vi "Begin.vi"(8 "error in":errorcluster) -> (0 "error out":errorcluster)   [LabVIEW 2019]
doc: "Called before other user functions, this VI is expected to open initial I/O refnums, load in file data, and do all program initialization. Notice that the <B>error out</B> terminal is simply used for data flow. Wiring it to other structures or subVIs ensures that this VI runs first."
uses:
  <vilib>/Rock Robotics/WPI/DriverStation/WPI_DriverStationRobotMode2.ctl
  <vilib>/Rock Robotics/WPI/ThirdParty/JAS_Junk/TrajLib/Translation2d_Create.vi
  Robot Global Data.vi
  <vilib>/Rock Robotics/Network Tables/NT Write String Array.vi
  <vilib>/Rock Robotics/WPI/ThirdParty/JAS_Junk/TrajLib/Trajectory_Library.lvlib
panel:
  in  "Tab Control":T1(tab)
  # "Instructions:\nThis should create a path, show the data on the various tabs and optionally write the motor demands and expected results to a file for use on a a robot..\n1) Enter robot data on Robot Data Tab\n2) Define your path definitions.\n3) Define the time increment.  0.020 is chosen since that matches the normal loop time.\n4) Press calculate path.  If a good path was calculated it will be displayed on the Tank Data tab, and the Ready to Execute will indicate execution can begin.\nThe path can be recalculated many times before selecting execute.\n\nTo write to a file.\n5) Select the file name\n6) This example uses \"steps\", sequential numbers for inclusion into a list based autonomous routine.  Including the step number if optional.\n7) This uses command numbers to indicate first, last, and intermediate steps.  This allows some simplification of the execution routine.  It\nalso allows the path to be executed backwards if desired.  The command numbers are changeable.\n8) Press \"Create Command List\".\n\nNotes:\n- PC robot simulataion is disabled in this program.  The code is still there if you want to restore it and try it out.  Use one of the other test programs \nto simulate the path on a PC.\n- The path generation logic doesn't account distribution of speed to the left and right wheels.  As a result the maximum speed can be exceeded.\nIf this happens, but Path Speed > Max light will light and Ready to Execute will not light.  Lower the maximum speed in the Robot Data tab\nand recalulate the path.\n- 2019 playing field size - width: 26 ft 11.25 In = 323.25 in , length: 52 ft 5.25 in = 629.25 in  (I didn't verify this for the 2020 version.)"
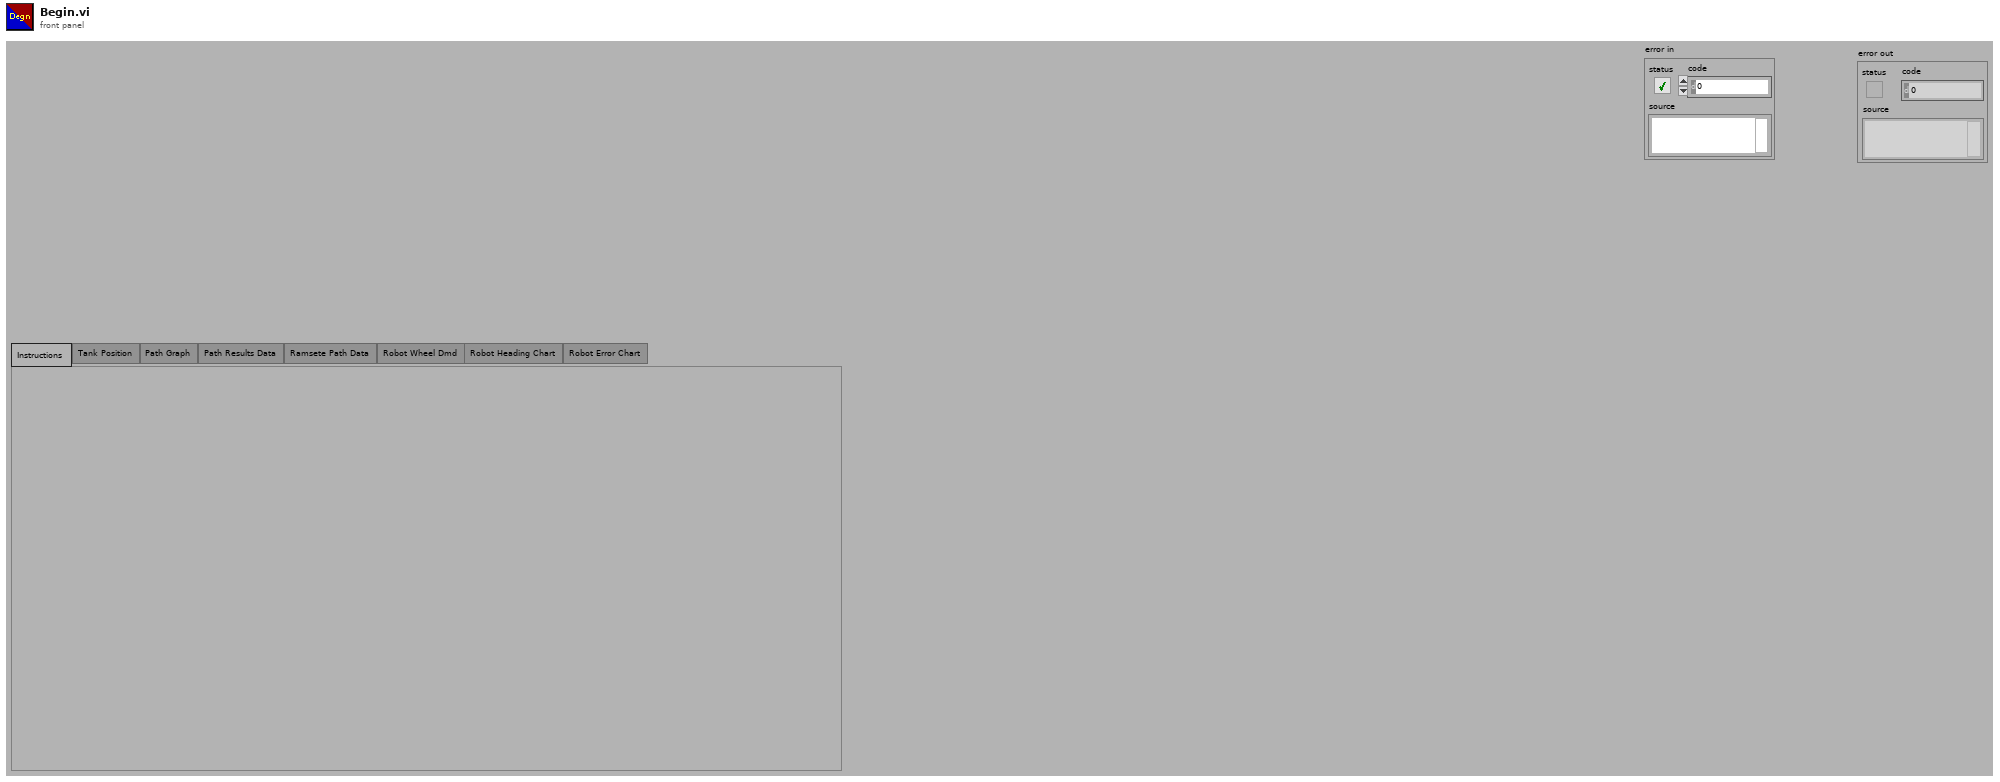
[diagram p1: front panel]
types:
  T1 = enum32{"Instructions", "Tank Position", "Path Graph", "Path Results Data", "Ramsete Path Data", "Robot Wheel Dmd", "Robot Heading Chart", "Robot Error Chart"}
  T2 = typedef "WPI_DriverStationRobotMode2.ctl" = enum16{"Autonomous Disabled", "Autonomous Enabled", "Teleop Disabled", "Teleop Enabled", "Disconnected", "Finish", "Test Disabled", "Test Enabled", "Emergency Stopped"}
  T3 = typedef "Trajectory_Library.lvlib/POSE2D.ctl" = cluster{"TRANSLATION":T4, "ROTATION":T5}
  T4 = typedef "Trajectory_Library.lvlib/TRANSLATION2D.ctl" = cluster{"X":dbl, "Y":dbl}
  T5 = typedef "Trajectory_Library.lvlib/ROTATION2D.ctl" = cluster{"VALUE":dbl, "COS":dbl, "SIN":dbl}
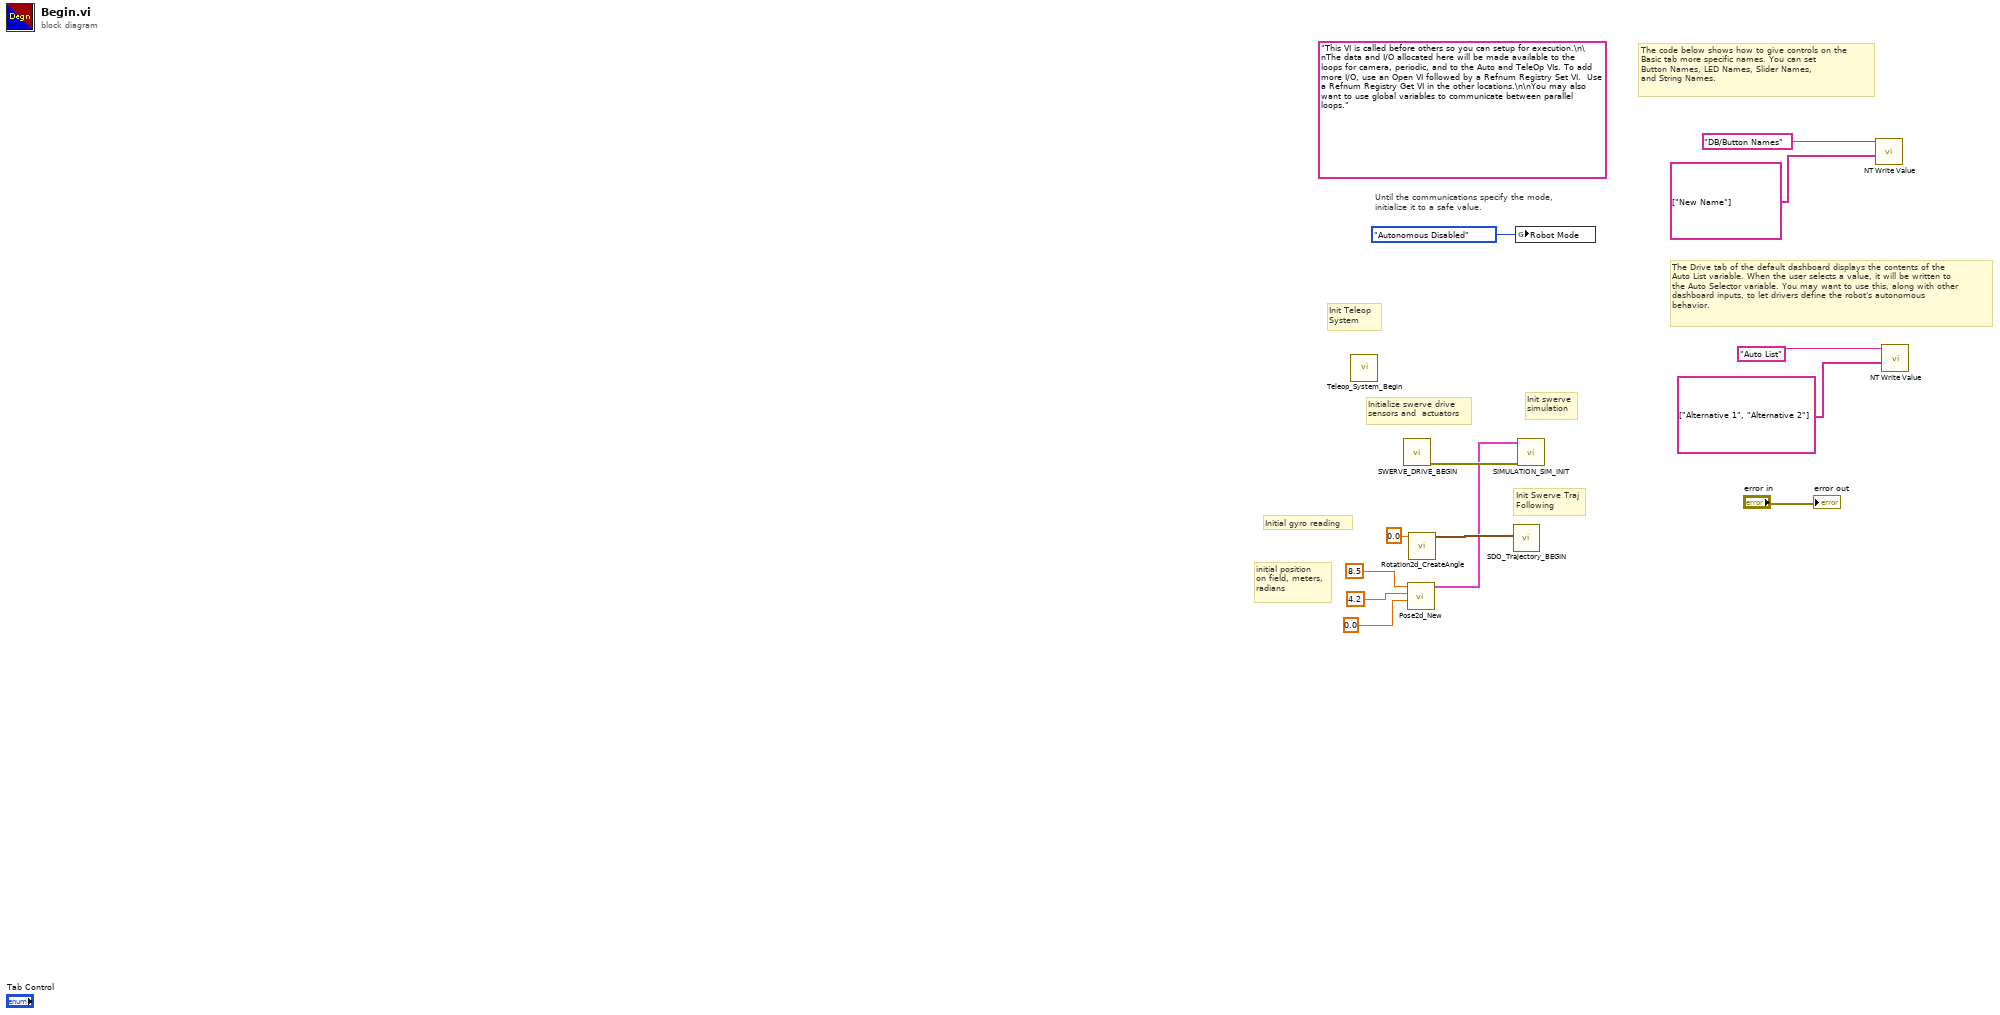
[diagram p0: block diagram]
diagram:
  (unwired) "This VI is called before others so you can setup for execution.\n\nThe data and I/O allocated here will be made available to the loops for camera, periodic, and to the Auto and TeleOp VIs. To add more I/O, use an Open VI followed by a Refnum Registry Set VI.  Use a Refnum Registry Get VI in the other locations.\n\nYou may also want to use global variables to communicate between parallel loops."
  # "Init swerve\nsimulation"
  # "Initial gyro reading"
  # "Init Teleop \nSystem"
  # "Init Swerve Traj\nFollowing"
  # "Initialize swerve drive\nsensors and  actuators"
  # "initial position\non field, meters,\nradians"
  # "The Drive tab of the default dashboard displays the contents of the\nAuto List variable. When the user selects a value, it will be written to\nthe Auto Selector variable. You may want to use this, along with other\ndashboard inputs, to let drivers define the robot's autonomous\nbehavior."
  # "The code below shows how to give controls on the\nBasic tab more specific names. You can set\nButton Names, LED Names, Slider Names,\nand String Names."
  # "Until the communications specify the mode,\ninitialize it to a safe value."
  n1 = call "Teleop_System_Begin.vi"() -> ()  [unwired: 12 in]
  n2 = call "SWERVE_DRIVE_BEGIN.vi"() -> ("error out"=w2:errorcluster)  [unwired: 11 in]
  n3 = call <vilib>:"Pose2d_New.vi"("Heading"=0.0, "Y"=4.2, "X"=8.5) -> ("out POSe"=w1:T3)  [unwired: 8 in]
  n4 = call <vilib>:"Rotation2d_CreateAngle.vi"("Angle"=0.0) -> ("ROTATION"=w4:T5)  [unwired: 10 in]
  n5 = call "SDO_Trajectory_BEGIN.vi"("gyroAngle"=w4) -> ()  [unwired: 11 in]
  n6 = global write "Robot Global Data.vi" "Robot Mode"(WPI_DriverStationRobotMode2."Autonomous Disabled" ("Robot Mode")) -> ()
  n7 = call "SIMULATION_SIM_INIT.vi"("error in (no error)"=w2, "Initial Robot Position"=w1) -> ()  [unwired: 9 in, 1 out]
  n8 = call-poly <vilib>:"NT Write Value.vi"("value"=string[] ["New Name"], "name"="DB/Button Names" ("Name")) -> ()  [unwired: 9 in, 1 out]
  n9 = call-poly <vilib>:"NT Write Value.vi"("value"=string[] ["Alternative 1", "Alternative 2"] ("String Array"), "name"="Auto List" ("Name")) -> ()  [unwired: 9 in, 1 out]
  "error out" <- "error in"
